vi "Trigger Delay Tracking.vi"(2 "Delay Data FIFO":refnum<k21>, 5 "conditioned start trigger":bool, 9 "unconditioned start trigger":bool, 11 "enable":bool) -> (14 "ready for input":bool)   [LabVIEW 2018, in "GettingStarted_5774_FPGA.lvlib"]
doc: "Counts the cycle delay between a rising edge on the <B>conditioned start trigger</B> input and the last rising edge on the <B>unconditioned start trigger</B> input. If the <B>enable</B> input is true, then the cycle delay value is written into the <B>Delay Data FIFO</B> FIFO. The <B>ready for input</B> output returns the ready for input output of the FIFO, or true if the <B>enable</B> input is false."
uses:
  <vilib>/rvi/DataTransferAndStorage/Container/Common/niFpgaContainerExecOnDevCompGetState.vi
  <vilib>/rvi/Emulation/niFpgaEmulationIsFPGAContextNoSignature.vi
  <vilib>/rvi/Emulation/niFpgaSctlEmulationGetInTimedLoop.vi
  <vilib>/rvi/errors/niFpgaSetErrorForExecOnDevCompSimple.vi
  <vilib>/rvi/eio/common/nirviEmuReportErrorAndStop.vi
  <vilib>/rvi/DataTransferAndStorage/Container/Common/niFpgaContainerGetUniqueNameForEmu.vi
  <vilib>/rvi/FIFO/Fifo_Resource/nirvififoEmulationSetSize.vi
  <vilib>/rvi/FIFO/Fifo_Resource/nirviFifoEmulationQueueMgr.vi
  <instcachedir>/0/nirviFifoEmulationQueueMgr_E5CAEC123FF24DC58D834DCA3CDAA9B5.lvgen/nirviFifoEmulationQueueMgr_E5CAEC123FF24DC58D834DCA3CDAA9B5_009.vi
  <vilib>/rvi/FIFO/Fifo_Resource/nirvififoEmulationDetermineInputValidOut.vi
  <vilib>/rvi/FIFO/Fifo_Resource/nirvififoEmulationCreateLock.vi
  <vilib>/rvi/Emulation/niFpgaProcessEmulError.vi
  <vilib>/rvi/FIFO/Fifo_Resource/nirvififoEmulationObtainLock.vi
  <vilib>/rvi/FIFO/Fifo_Resource/nirvififoEmulationReleaseLock.vi
  <vilib>/rvi/occurrence/nirviWaitOnOccurrenceBase.vi
  <vilib>/rvi/errors/nirviReportUnexpectedCaseInternalError.vi
  <vilib>/rvi/errors/nirviReportUnexpectedCaseInternalError (U32).vi
  <vilib>/Utility/error.llb/Clear Errors.vi
  <vilib>/rvi/interface/RandomDataEmulation/niFpgaRandomDataHandleErrors.vi
  <instrlib>/_niInstr/Basic Elements/v1/FPGA/Private/Count Up U32.vi
  <vilib>/rvi/DataTransferAndStorage/Container/XNode/niFpgaContainer.xnode
  <vilib>/rvi/FIFO/Fifo_Resource/niFpgaFifoEmulationRefIn.vi
  GettingStarted_5774_FPGA.lvlib
  <instrlib>/_niInstr/Basic Elements/v1/FPGA/niInstr Basic Elements v1 FPGA.lvlib
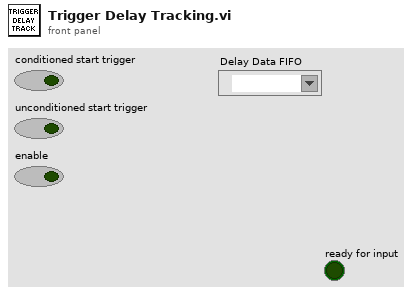
[diagram p1: front panel]
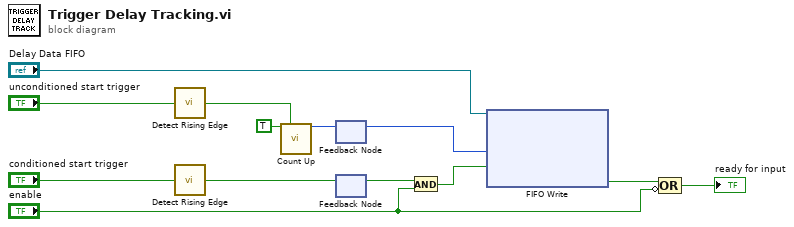
[diagram p0: block diagram]
diagram:
  n1 = call <instrlib>:"Detect Rising Edge.vi"("signal"="unconditioned start trigger") -> ("edge detected"=w8:bool)  [unwired: 14 in]
  n2 = call <instrlib>:"Detect Rising Edge.vi"("signal"="conditioned start trigger") -> ("edge detected"=w9:bool)  [unwired: 14 in]
  n3 = call-poly <instrlib>:"Count Up.vi"("increment"=TRUE, "reset"=w8) -> ("count out"=w11:u32)  [unwired: 13 in]
  n4 = feedback-in #1(w11) -> ()
  n5 = feedback #1() -> (w4:u32)  [unwired: 1 in]
  n6 = feedback #2() -> (w7:bool)  [unwired: 1 in]
  n7 = feedback-in #2(w9) -> ()
  n8 = And(x=w7, y="enable") -> (x .and. y?=w5:bool)
  n9 = xnode "FIFO Write"("Element"=w4, "Input Valid"=w5, "FIFO In"="Delay Data FIFO") -> ("Ready for Input"=w3:bool)  [unwired: 1 out]
  n10 = Compound Arithmetic op=OR(w3, invert "enable") -> (→"ready for input":bool)
